vi "XmitMIMICCommand.vi"(2 "error in (no error)":errorcluster {"code" format="%.0x"}, 3 "HWHSflag":bool=TRUE, 4 "Command array":u8[](array[numeric]) format="%x", 5 "VISA resource name":refnum<visa-resource-name>="COM1") -> (0 "error out":errorcluster, 1 "VISA resource name Out":refnum<visa-resource-name>)   [LabVIEW 2014]
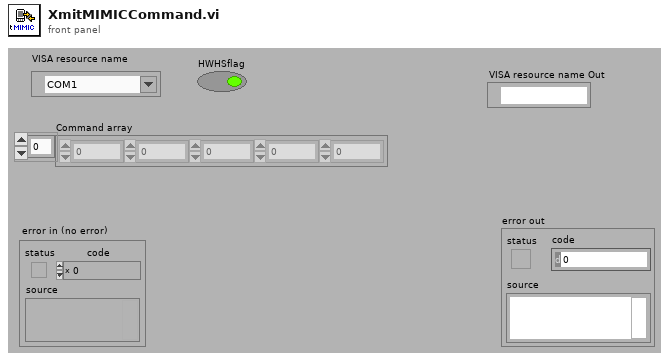
[diagram p1: front panel]
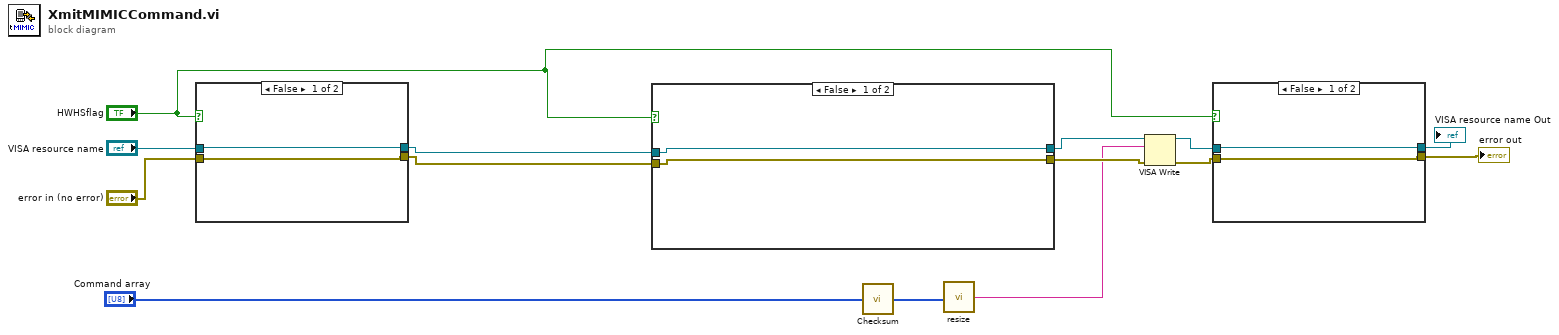
[diagram p0: block diagram]
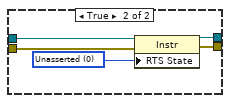
[diagram p2: hidden frame]
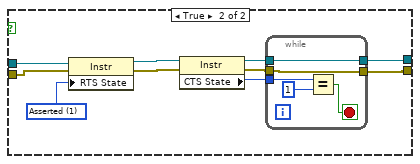
[diagram p3: hidden frame]
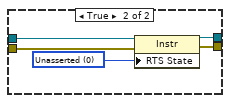
[diagram p4: hidden frame]
diagram:
  n1 = case shown="False" "HWHSflag" {
    tunnel: "VISA resource name" -> [w16 w20]
    tunnel: "error in (no error)" -> [w15 w19]
    tunnel: [w16 w18] -> w2
    tunnel: [w15 w17] -> w1
    frame False {
    }
    frame True {
      w21 = i16 0 items=["Unknown"=-1, "Unasserted"=0, "Asserted"=1] ("Serial Settings:Modem Line Settings:Line RTS State")
      n2 = property class="Instr"(reference=w20, error in=w19, "RTS State"=w21) -> (reference out=w18:refnum<visa-resource-name>, error out=w17:errorcluster)
    }
  }
  n3 = case shown="False" "HWHSflag" {
    tunnel: [w23 w27] -> w11
    tunnel: [w22 w26] -> w12
    tunnel: w2 -> [w23 w25]
    tunnel: w1 -> [w22 w24]
    frame False {
    }
    frame True {
      w33 = i16 1 items=["Unknown"=-1, "Unasserted"=0, "Asserted"=1] ("Serial Settings:Modem Line Settings:Line RTS State")
      n4 = property class="Instr"(reference=w25, error in=w24, "RTS State"=w33) -> (reference out=w32:refnum<visa-resource-name>, error out=w31:errorcluster)
      n5 = property class="Instr"(reference=w32, error in=w31) -> (reference out=w29:refnum<visa-resource-name>, error out=w28:errorcluster, "CTS State"=w30:i16)
      n6 = while {
        tunnel: w30 -> [w38]
        tunnel: w29 -> [w34]
        tunnel: [w35] -> w26
        tunnel: w28 -> [w35]
        tunnel: [w34] -> w27
        stop <- w36 stop-if-true
        n7 = Equal?(x=w38, y=i16 1) -> (x = y?=w36:bool)
      }
    }
  }
  n8 = call "Checksum.vi"("input array"="Command array") -> ("output array"=w4:u8[])
  n9 = call "resize.vi"("Array"=w4) -> ("MIMIC_CMD"=w3:string)
  n10 = VISA Write(VISA resource name=w11, write buffer=w3, error in (no error)=w12) -> (VISA resource name out=w9:refnum<visa-resource-name>, error out=w10:errorcluster)  [unwired: 1 out]
  n11 = case shown="False" "HWHSflag" {
    tunnel: w9 -> [w40 w44]
    tunnel: w10 -> [w39 w43]
    tunnel: [w40 w42] -> w5
    tunnel: [w39 w41] -> w8
    frame False {
    }
    frame True {
      w45 = i16 0 items=["Unknown"=-1, "Unasserted"=0, "Asserted"=1] ("Serial Settings:Modem Line Settings:Line RTS State")
      n12 = property class="Instr"(reference=w44, error in=w43, "RTS State"=w45) -> (reference out=w42:refnum<visa-resource-name>, error out=w41:errorcluster)
    }
  }
  "error out" <- w8
  "VISA resource name Out" <- w5
